vi "makeFitPlotCommands.vi"(5 "Fit Zmin":dbl=500.0 min=0.0, 6 "plotInfoArray":T1(array[cluster]), 7 "Fit Zmax":dbl=500.0 min=0.0, 9 "BL Targets":T2[](array[typedef]) {"n" min=0.02 max=0.5 step=0.01 format="%.2f"}, 10 "Coefficients":cluster{"No d0":T3, "with d0":T3}, 11 "Zref":dbl=508.0 min=0.0) -> (1 "UnderlayPlotSeries":string[](array[string])=["fitmin = 100, fitmax=550, zref=508, d=16.2, n=0.121, clippedpowerlaw(x) w line ls 1 lw 10 lc rgb \"gray25\" title 'fit with displacement'", "fitmin = 100, fitmax=550, zref=508, d=0, n=0.133, clippedpowerlaw(x) w line ls 1 lw 8 lc rgb \"gray50\" title 'zero displacement fit'", "zref=508, d=0, n=0.170, powerlaw(x) w line ls 0 lw 1 lc rgb \"gray75\" title 'target power law'"], 2 "Pre-plot Injection":string, 3 "BasicsVisible":bool[](array[boolean]))   [LabVIEW 2014]
uses:
  PowerLaw.ctl
  BLTarget.ctl
  at.ctl
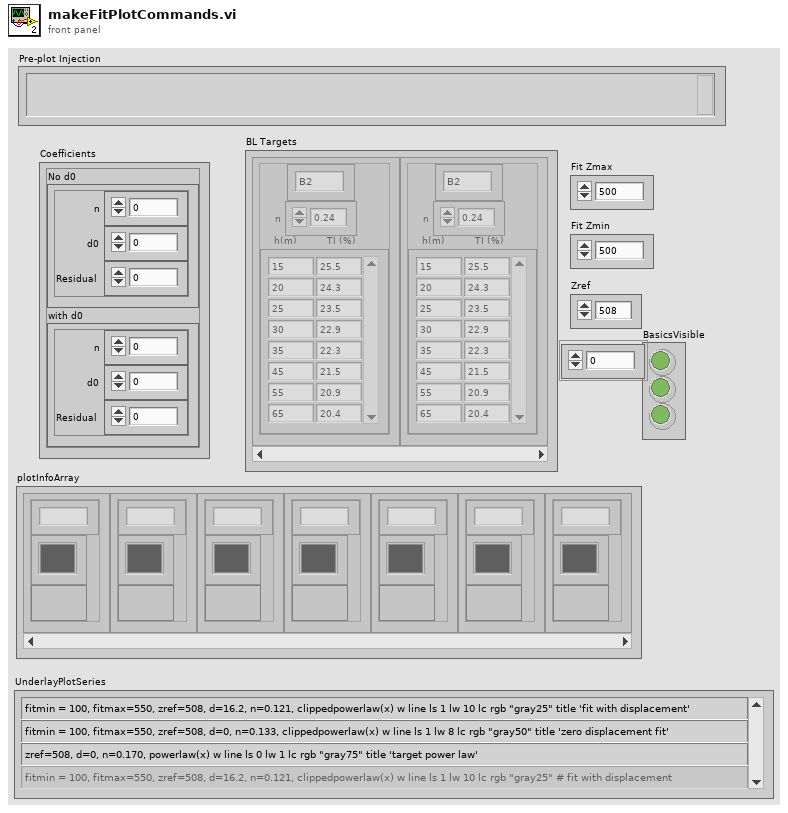
[diagram p1: front panel]
types:
  T1 = cluster{"Plot Name":string, "Plot.Plot Color":u32, "Plot.Visible?":bool}[]
  T2 = typedef "BLTarget.ctl" = cluster{"Code":string, "TI Profile (FS)":dbl[][], "n":dbl}
  T3 = typedef "PowerLaw.ctl" = cluster{"n":dbl, "d0":dbl, "Residual":dbl}
  T4 = typedef "at.ctl" = cluster{"XcoordSys":string, "YcoordSys":string, "Xvalue":dbl, "Yvalue":dbl}
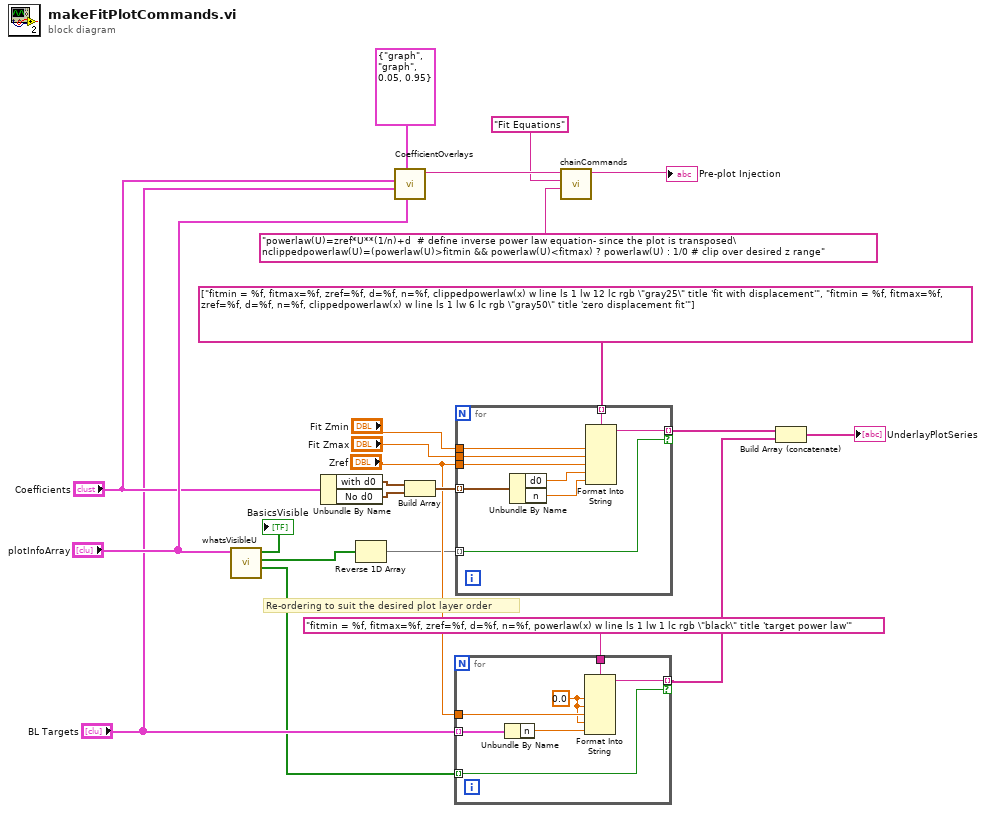
[diagram p0: block diagram]
diagram:
  # "Re-ordering to suit the desired plot layer order"
  n1 = call "whatsVisibleU.vi"("UplotInfoArray"="plotInfoArray") -> ("Targets Visible"=w4:bool[], "Fits Visible"=w2:bool[], "BasicsVisible"=→"BasicsVisible":bool[])  [unwired: 8 in]
  n2 = Unbundle By Name("Coefficients") -> ("with d0"=w22:T3, "No d0"=w21:T3)
  n3 = Reverse 1D Array(array=w2) -> (reversed array=w3:bool[])
  n4 = call "CoefficientOverlays.vi"("plotInfoArray"="plotInfoArray", "\"At\" location"=T4 {"XcoordSys"="graph", "YcoordSys"="graph", "Xvalue"=0.05, "Yvalue"=0.95} ("\"At\" location"), "BL Targets"="BL Targets", "Coefficients"="Coefficients") -> ("gnuplotOut"=w17:string)  [unwired: 7 in]
  n5 = Build Array(w22, w21) -> (w19:T3[])
  n6 = for {
    tunnel: "fitmin = %f, fitmax=%f, zref=%f, d=%f, n=%f, powerlaw(x) w line ls 1 lw 1 lc rgb \"black\" title 'target power law'" ("String") -> [w30]
    tunnel: "BL Targets" -> [w29] mode=indexing
    tunnel: [w28] -> w8 mode=indexing if=w24
    tunnel: w4 -> [w24] mode=indexing
    tunnel: "Zref" -> [w27]
    w26 = 0.0 ("input 1")
    n7 = Unbundle By Name(w29) -> ("n"=w25:dbl)
    n8 = Format Into String(format string=w30, w26, w26, w27, w26, w25) -> (resulting string=w28:string)  [unwired: 2 in, 1 out]
  }
  n9 = for {
    tunnel: string[] ["fitmin = %f, fitmax=%f, zref=%f, d=%f, n=%f, clippedpowerlaw(x) w line ls 1 lw 12 lc rgb \"gray25\" title 'fit with displacement'", "fitmin = %f, fitmax=%f, zref=%f, d=%f, n=%f, clippedpowerlaw(x) w line ls 1 lw 6 lc rgb \"gray50\" title 'zero displacement fit'"] ("UnderlayPlotSeries 2") -> [w39] mode=indexing
    tunnel: w19 -> [w38] mode=indexing
    tunnel: "Fit Zmin" -> [w37]
    tunnel: "Fit Zmax" -> [w36]
    tunnel: [w33] -> w18 mode=indexing if=w31
    tunnel: w3 -> [w31] mode=indexing
    tunnel: "Zref" -> [w32]
    n10 = Unbundle By Name(w38) -> ("d0"=w35:dbl, "n"=w34:dbl)
    n11 = Format Into String(format string=w39, w37, w36, w32, w35, w34) -> (resulting string=w33:string)  [unwired: 2 in, 1 out]
  }
  n12 = call "chainCommands.vi"("Command"="powerlaw(U)=zref*U**(1/n)+d  # define inverse power law equation- since the plot is transposed\nclippedpowerlaw(U)=(powerlaw(U)>fitmin && powerlaw(U)<fitmax) ? powerlaw(U) : 1/0 # clip over desired z range" ("FitEquations"), "Comments"="Fit Equations", "StringIn"=w17) -> ("StringOut"=→"Pre-plot Injection":string)  [unwired: 8 in]
  n13 = Build Array (concatenate)(w18, w8) -> (→"UnderlayPlotSeries":string[])
